vi "POST File Upload Example.vi"() -> ()   [LabVIEW 2017]
uses:
  <vilib>/httpClient/MultipartData.ctl
  <vilib>/addons/_JKI.lib/REST Client/classes/REST Client/REST Client.lvclass
  <vilib>/httpClient/LabVIEWHTTPClient.lvlib
panel:
  in  "Authentication":cluster{"Username":string, "Password":string}
  out "Status String":string
  out "Status Code":u16
  out "Response body":string
  in  "API Endpoint":string="upload"
  out "error out":errorcluster
  in  "FIlepath":path=path "D:/upwork/Labview-REST-API/labview-source/payload.png"
  in  "API Base Url":string="https://luferau.free.beeceptor.com/"
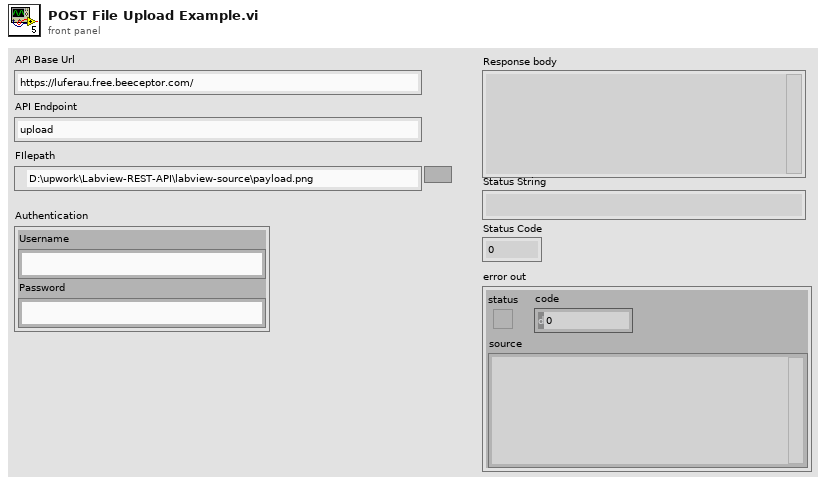
[diagram p1: front panel]
types:
  T1 = typedef "LabVIEWHTTPClient.lvlib/MultipartData.ctl" = cluster{"Name":string, "Value":string, "File":path, "Filename":string, "MIME type":string}
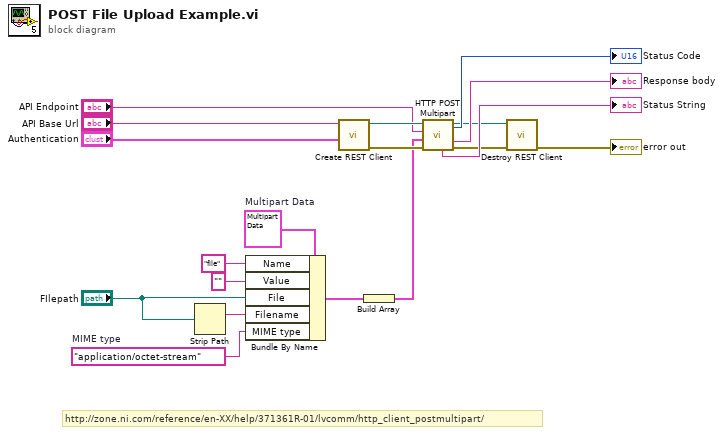
[diagram p0: block diagram]
diagram:
  w13 = "application/octet-stream"  # MIME type
  w18 = T1 {"Name"="", "Value"="", "File"=path "", "Filename"="", "MIME type"="application/octet-stream"}  # Multipart Data
  # "http://zone.ni.com/reference/en-XX/help/371361R-01/lvcomm/http_client_postmultipart/"
  n1 = Strip Path(path="FIlepath") -> (name=w14:string)  [unwired: 1 out]
  n2 = Bundle By Name(cluster=w18, "Name"="file", "Value"="", "File"="FIlepath", "Filename"=w14, "MIME type"=w13) -> (w10:T1)
  n3 = call <vilib>:"Create REST Client.vi"("Authentication"="Authentication", "Base URL"="API Base Url") -> ("error out"=w11:errorcluster, "REST Client out"=w12:refnum<class "REST Client.lvclass">)  [unwired: 8 in]
  n4 = Build Array(w10) -> (w2:T1[])
  n5 = call-dynamic "HTTP POST Multipart.vi"("error in (no error)"=w11, "Multipart Post data"=w2, "Path"="API Endpoint", "REST Client in"=w12) -> ("error out"=w4:errorcluster, "Response body"=→"Response body":string, "REST Client out"=w5:refnum<class "REST Client.lvclass">, "Status String"=→"Status String":string, "Status Code"=→"Status Code":u16)  [unwired: 2 in, 1 out]
  n6 = call-dynamic "Destroy REST Client.vi"("error in (no error)"=w4, "REST Client in"=w5) -> ("error out"=→"error out":errorcluster)  [unwired: 9 in]
